vi "Decrypt Play Item.vi"(4 "Encrypted Play Item":string) -> (1 "Play Item":T1)   [LabVIEW 2020, in "AoC 2022.lvlib"]
uses:
  Play Item.ctl
  AoC 2022.lvlib
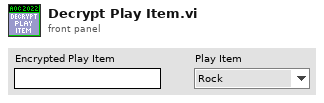
[diagram p1: front panel]
types:
  T1 = typedef "AoC 2022.lvlib/Play Item.ctl" = enum16{"Rock", "Paper", "Scissor"}
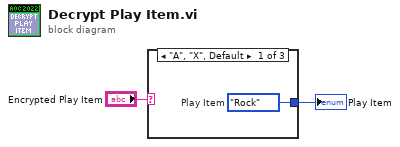
[diagram p0: block diagram]
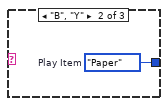
[diagram p2: hidden frame]
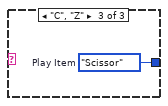
[diagram p3: hidden frame]
diagram:
  n1 = case shown="\"A\", \"X\", Default" "Encrypted Play Item" {
    tunnel: [w3 w4 w5] -> w2
    frame "A", "X", Default {
      w3 = Play_Item."Rock"  # Play Item
    }
    frame "B", "Y" {
      w4 = Play_Item."Paper"  # Play Item
    }
    frame "C", "Z" {
      w5 = Play_Item."Scissor"  # Play Item
    }
  }
  "Play Item" <- w2
